vi "CommandCycle.vi"(8 "Gripper Value R":dbl, 9 "Gripper Value L":dbl, 10 "Elevator Value":dbl, 11 "Teir Selection":T2) -> (3 "appended array":cluster{"States":T1, "Close":dbl[]}[](array[cluster]))   [LabVIEW 2014, in "Elevator System.lvlib"]
uses:
  Elevator System.lvlib
  Typedef/ControllerStates.ctl
  Typedef/TeirNumber.ctl
panel:
  out "appended array":cluster{"States":T1, "Numeric":dbl}[](array[cluster])
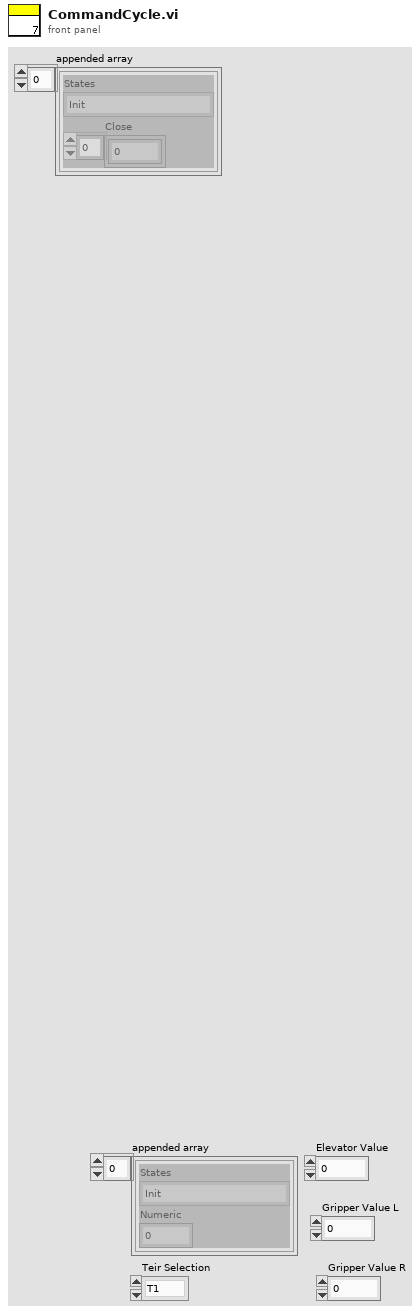
[diagram p1: front panel]
types:
  T1 = typedef "Elevator System.lvlib/ControllerStates.ctl" = enum16{"Init", "Set Elevator SP", "Set Gripper SP", "Wait For Elevator", "Wait For Gripper", ""}
  T2 = typedef "Elevator System.lvlib/TeirNumber.ctl" = enum16{"T1", "T2", "T3", "T4", "T5", "T6"}
  T3 = typedef "Elevator System.lvlib/GripperNotifierType.ctl" = cluster{"SP Left":dbl, "SP Right":dbl}
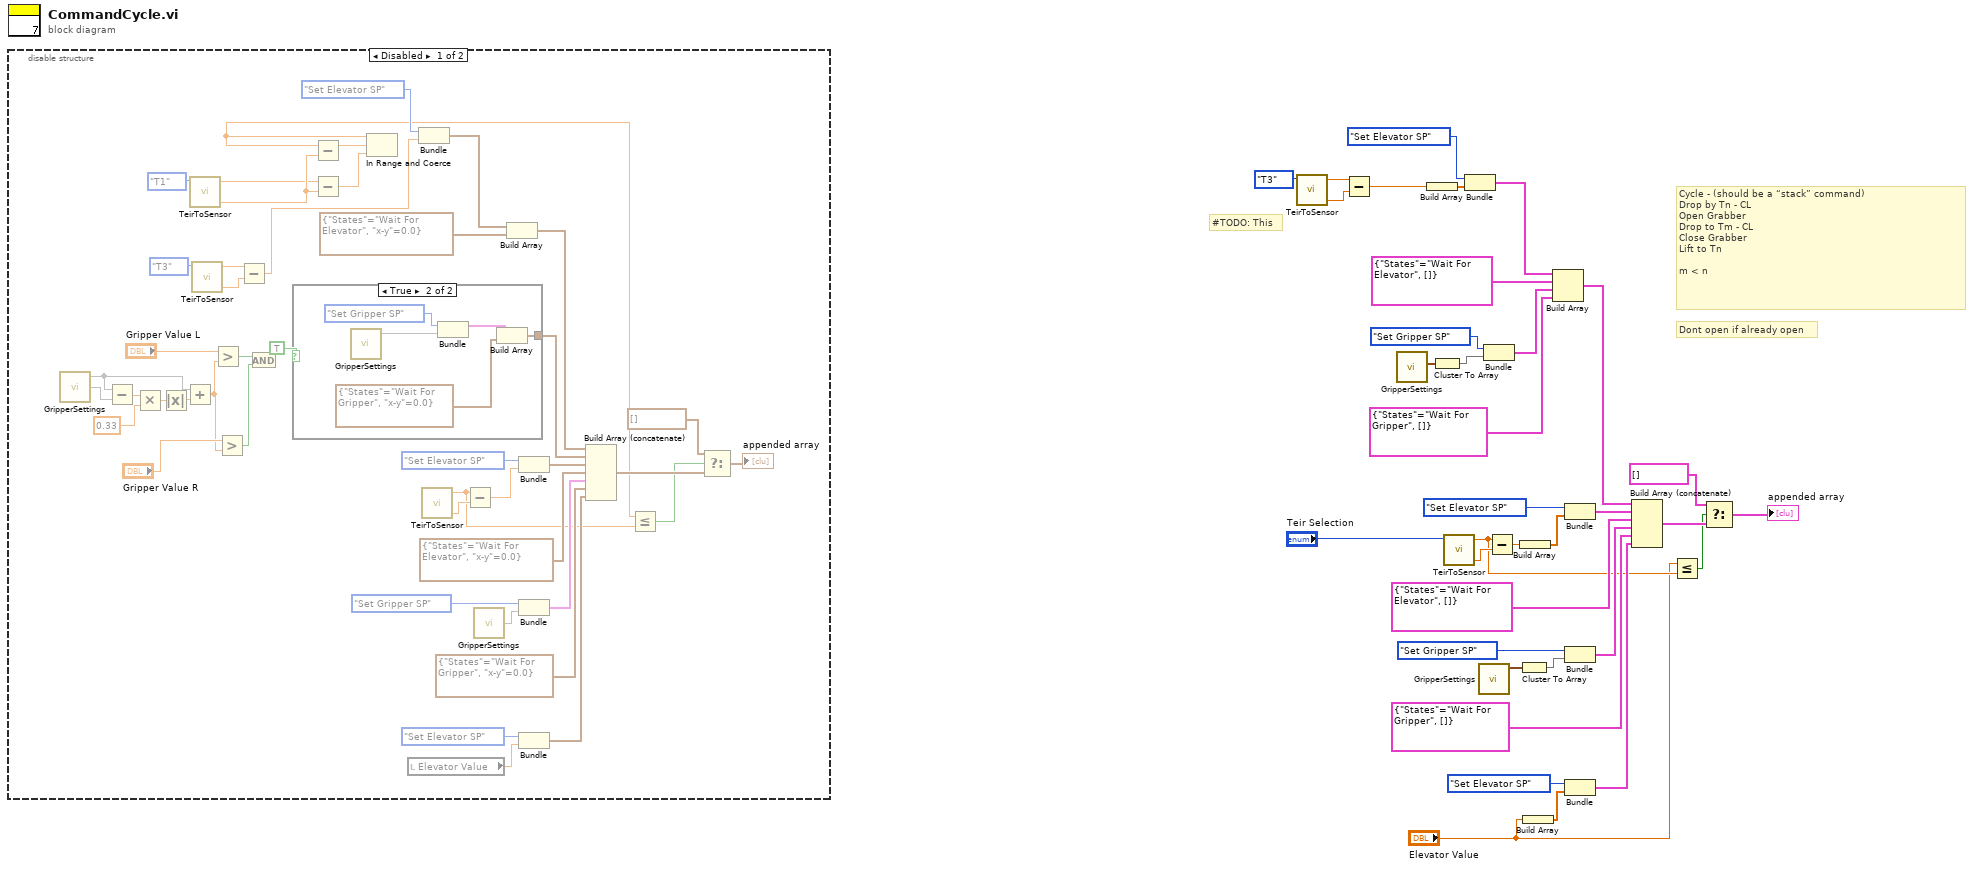
[diagram p0: block diagram]
diagram:
  # "#TODO: This"
  # "Dont open if already open"
  # "Cycle - (should be a “stack” command)\nDrop by Tn - CL\nOpen Grabber\nDrop to Tm - CL\nClose Grabber\nLift to Tn\n\nm < n"
  n1 = disable-structure shown="Disabled" {
    frame Disabled {
      n2 = call "GripperSettings.vi"() -> (2:w66, 3:w61)  [unwired: 3 in]
      n3 = Subtract(x=w66, y=w61) -> (x-y=w62:dbl)
      n4 = Multiply(x=w62, y=0.33) -> (x*y=w64:dbl)
      n5 = Absolute Value(x=w64) -> (abs(x)=w65:dbl)
      n6 = Add(x=w66, y=w65) -> (x+y=w48:dbl)
      n7 = call "TeirToSensor.vi"("Enum"=TeirNumber."T1") -> ("T1"=w67:dbl, "CL"=w68:dbl)  [unwired: 3 in, 3 out]
      n8 = call "TeirToSensor.vi"("Enum"=TeirNumber."T3") -> ("T1"=w38:dbl, "CL"=w37:dbl)  [unwired: 3 in, 3 out]
      n9 = Greater?(x="Gripper Value L", y=w48) -> (0:w53:bool)
      n10 = Greater?(x="Gripper Value R", y=w48) -> (0:w47:bool)
      n11 = Subtract(x=w38, y=w37) -> (x-y=w36:dbl)
      n12 = And(x=w53, y=w47) -> ()  [unwired: 1 out]
      n13 = case shown="True" TRUE {
        tunnel: [_ w83] -> w54
        frame False {
        }
        frame True {
          n14 = call "GripperSettings.vi"() -> (2:w84)  [unwired: 4 in]
          n15 = Bundle("States"=ControllerStates."Set Gripper SP", w84) -> (w82:cluster{"States":T1, void})  [unwired: 1 in]
          n16 = Build Array(w82, cluster{"States":T1, "x-y":dbl} {"States"=enum."Wait For Gripper", "x-y"=0.0}) -> (w83:cluster{"States":T1, "x-y":dbl}[])
        }
      }
      n17 = Subtract(x=w67, y=w68) -> (x-y=w57:dbl)
      n18 = local read "Elevator Value"() -> (w50:dbl)
      n19 = Bundle("States"=ControllerStates."Set Elevator SP", w36) -> (w56:cluster{"States":T1, dbl})  [unwired: 1 in]
      n20 = call "TeirToSensor.vi"() -> ("Enum"=w51:T2, "T1"=w41:dbl, "CL"=w78:dbl)  [unwired: 3 in, 3 out]
      n21 = Subtract(x=w41, y=w78) -> (x-y=w77:dbl)
      n22 = call "GripperSettings.vi"() -> (3:w72)  [unwired: 4 in]
      n23 = Build Array(w56, cluster{"States":T1, "x-y":dbl} {"States"=enum."Wait For Elevator", "x-y"=0.0}) -> (w69:cluster{"States":T1, "x-y":dbl}[])
      n24 = Bundle("States"=ControllerStates."Set Elevator SP", w77) -> (w75:cluster{"States":T1, dbl})  [unwired: 1 in]
      n25 = Bundle("States"=ControllerStates."Set Gripper SP", w72) -> (w73:cluster{"States":T1, void})  [unwired: 1 in]
      n26 = Bundle("States"=ControllerStates."Set Elevator SP", "Elevator Value"=w50) -> (w80:cluster{"States":T1, "Elevator Value":dbl})  [unwired: 1 in]
      n27 = Build Array (concatenate)(w69, w54, w75, cluster{"States":T1, "x-y":dbl} {"States"=enum."Wait For Elevator", "x-y"=0.0}, w73, cluster{"States":T1, "x-y":dbl} {"States"=enum."Wait For Gripper", "x-y"=0.0}, w80) -> (w45:cluster{"States":T1, "Elevator Value":dbl}[])
      n28 = Subtract(x=w42, y=w68) -> (x-y=w58:dbl)
      n29 = In Range and Coerce(x=w58, lower limit=w57) -> (upper limit=w42:dbl)  [unwired: 2 out]
      n30 = Less Or Equal?(x=w42, y=w41) -> (x <= y?=w44:bool)
      n31 = Select(t=cluster{"States":T1, "Elevator Value":dbl}[] [], s=w44, f=w45) -> (s? t:f=→"appended array":cluster{"States":T1, "Elevator Value":dbl}[])
    }
    frame Enabled {
    }
  }
  n32 = call "TeirToSensor.vi"("Enum"=TeirNumber."T3") -> ("T1"=w10:dbl, "CL"=w9:dbl)  [unwired: 3 in, 3 out]
  n33 = Subtract(x=w10, y=w9) -> (x-y=w8:dbl)
  n34 = call "GripperSettings.vi"() -> ("Open"=w13:T3)  [unwired: 5 in, 3 out]
  n35 = Build Array(w8) -> (w14:dbl[])
  n36 = Cluster To Array(cluster=w13) -> (array=w12:dbl[])
  n37 = call "TeirToSensor.vi"("Enum"="Teir Selection") -> ("T1"=w2:dbl, "CL"=w33:dbl)  [unwired: 3 in, 3 out]
  n38 = Bundle("States"=ControllerStates."Set Elevator SP", w14) -> (w19:cluster{"States":T1, dbl[]})  [unwired: 1 in]
  n39 = call "GripperSettings.vi"() -> ("Close"=w24:T3)  [unwired: 5 in, 3 out]
  n40 = Bundle("States"=ControllerStates."Set Gripper SP", "Open"=w12) -> (w17:cluster{"States":T1, "Open":dbl[]})  [unwired: 1 in]
  n41 = Subtract(x=w2, y=w33) -> (x-y=w32:dbl)
  n42 = Cluster To Array(cluster=w24) -> (array=w23:dbl[])
  n43 = Build Array(w32) -> (w26:dbl[])
  n44 = Build Array("Elevator Value") -> (w21:dbl[])
  n45 = Build Array(w19, cluster{"States":T1, dbl[]} {"States"=enum."Wait For Elevator", []}, w17, cluster{"States":T1, dbl[]} {"States"=enum."Wait For Gripper", []}) -> (w27:cluster{"States":T1, "Open":dbl[]}[])
  n46 = Bundle("States"=ControllerStates."Set Elevator SP", w26) -> (w30:cluster{"States":T1, dbl[]})  [unwired: 1 in]
  n47 = Bundle("States"=ControllerStates."Set Gripper SP", "Close"=w23) -> (w28:cluster{"States":T1, "Close":dbl[]})  [unwired: 1 in]
  n48 = Bundle("States"=ControllerStates."Set Elevator SP", w21) -> (w35:cluster{"States":T1, dbl[]})  [unwired: 1 in]
  n49 = Build Array (concatenate)(w27, w30, cluster{"States":T1, dbl[]} {"States"=enum."Wait For Elevator", []}, w28, cluster{"States":T1, dbl[]} {"States"=enum."Wait For Gripper", []}, w35) -> (w6:cluster{"States":T1, "Close":dbl[]}[])
  n50 = Less Or Equal?(x="Elevator Value", y=w2) -> (x <= y?=w4:bool)
  n51 = Select(t=cluster{"States":T1, "Close":dbl[]}[] [], s=w4, f=w6) -> (s? t:f=→"appended array":cluster{"States":T1, "Close":dbl[]}[])
